vi "RMS.vi"(7 "SlaveID":u8=1, 8 "error in (no error)":errorcluster, 11 ".NET Refnum in":refnum<k24>) -> (0 "error out":errorcluster, 2 "Acc RMS":u16[](array[numeric]), 3 "reference out":refnum<k24>)   [LabVIEW 2017]
uses:
  dll/Modbus.dll
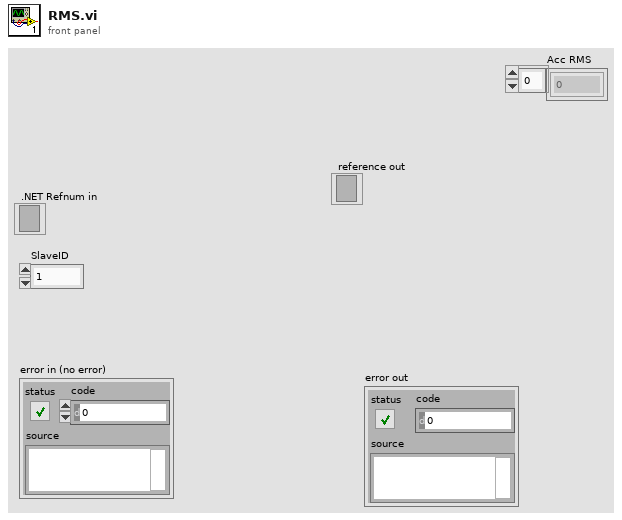
[diagram p1: front panel]
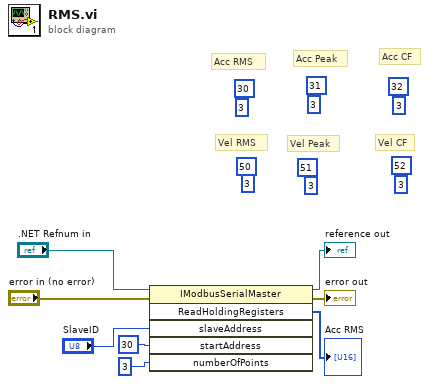
[diagram p0: block diagram]
diagram:
  (unwired) u16 3 ("numberOfPoints")
  (unwired) u16 3 ("numberOfPoints")
  (unwired) u16 52 ("startAddress")
  (unwired) u16 51 ("startAddress")
  (unwired) u16 3 ("numberOfPoints")
  (unwired) u16 50 ("startAddress")
  (unwired) u16 3 ("numberOfPoints")
  (unwired) u16 32 ("startAddress")
  (unwired) u16 3 ("numberOfPoints")
  (unwired) u16 31 ("startAddress")
  (unwired) u16 3 ("numberOfPoints")
  (unwired) u16 30 ("startAddress")
  # "Vel CF"
  # "Vel Peak"
  # "Vel RMS"
  # "Acc CF"
  # "Acc Peak"
  # "Acc RMS"
  n1 = invoke class="IModbusSerialMaster" method="ReadHoldingRegisters"(reference=".NET Refnum in", error in="error in (no error)", "slaveAddress"="SlaveID", "startAddress"=u16 30, "numberOfPoints"=u16 3) -> (reference out=→"reference out":refnum<k24>, error out=→"error out":errorcluster, "ReadHoldingRegisters"=→"Acc RMS":u16[])  [unwired: 1 in, 3 out]
